vi "apply channel changes.vi"(8 "error in":errorcluster, 9 "TBM channel in":refnum<class "TBM channel.lvclass">, 10 "TBM channel in":refnum<class "TBM channel.lvclass">, 11 "Tag Bus Web Interface configuration in":refnum<class "Tag Bus Web Interface configuration.lvclass">) -> (0 "error out":errorcluster, 3 "Tag Bus Web Interface configuration out":refnum<class "Tag Bus Web Interface configuration.lvclass">)   [LabVIEW 2013, in "Tag Bus Web Interface configuration.lvclass"]
uses:
  Tag Bus Web Interface configuration.lvclass
  <vilib>/NI/Tag Bus Module Framework/channel/TBM channel.lvclass
  Tag Bus Web Interface configuration.lvclass/Tag Bus Web Interface configuration.ctl
  <vilib>/NI/Tag Bus/tag/tag descriptor.lvclass/tag descriptor.ctl
  <vilib>/NI/Tag Bus/tag/read tag name.vi
  <vilib>/NI/Tag Bus/tag/tag descriptor.lvclass
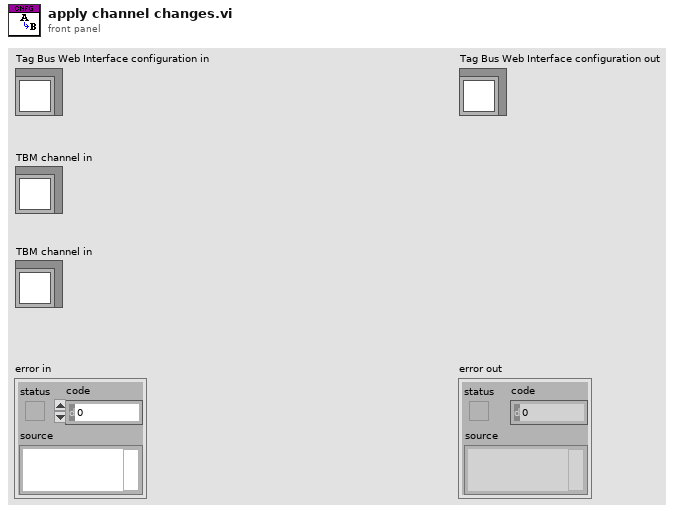
[diagram p1: front panel]
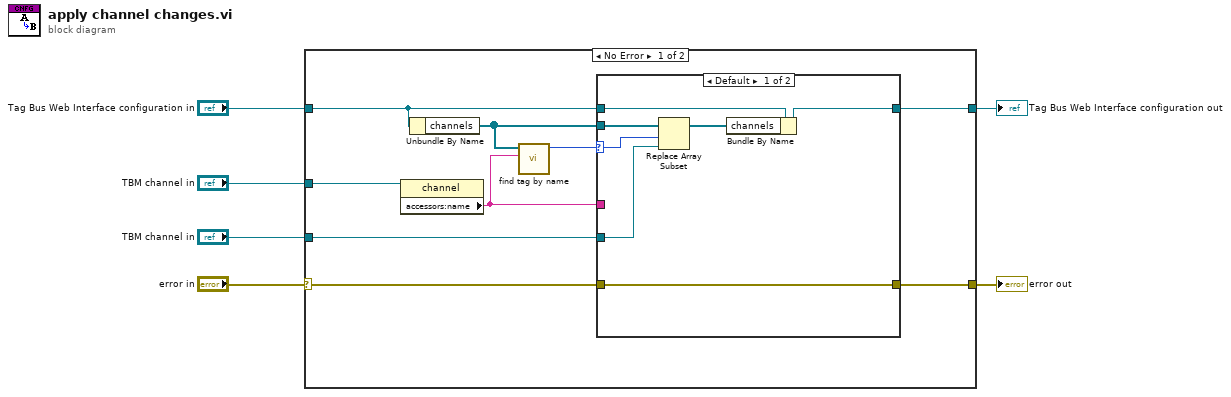
[diagram p0: block diagram]
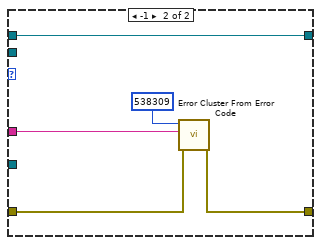
[diagram p2: hidden frame]
diagram:
  n1 = case shown="No Error" "error in" {
    selector: "error in" -> [w9 w29]
    tunnel: [w8 w29] -> w5
    tunnel: [w13 w28] -> w3
    tunnel: "Tag Bus Web Interface configuration in" -> [w14 w28]
    tunnel: "TBM channel in" -> [w15 _]
    tunnel: "TBM channel in" -> [w11 _]
    frame No Error {
      n2 = property class="channel"(reference=w15) -> ("accessors:name"=w10:string)  [unwired: 1 in, 2 out]
      n3 = Unbundle By Name(w14) -> ("channels"=w12:refnum<class "TBM channel.lvclass">[])
      n4 = call <vilib>:"find tag by name.vi"("name"=w10, "tags in"=w12) -> ("index"=w7:i32)  [unwired: 9 in]
      n5 = case shown="Default" w7 {
        selector: w7 -> [w20 _]
        tunnel: w14 -> [w22 w27]
        tunnel: [w19 w27] -> w13
        tunnel: w12 -> [w21 _]
        tunnel: w11 -> [w17 _]
        tunnel: w10 -> [_ w25]
        tunnel: w9 -> [w16 w24]
        tunnel: [w16 w23] -> w8
        frame Default {
          n6 = Replace Array Subset(array=w21, new element=w17, index=w20) -> (w18:refnum<class "TBM channel.lvclass">[])
          n7 = Bundle By Name(cluster=w22, "channels"=w18) -> (w19:refnum<class "Tag Bus Web Interface configuration.lvclass">)
        }
        frame -1 {
          n8 = call <vilib>:"Error Cluster From Error Code.vi"("error in (no error)"=w24, "error message (\"\")"=w25, "error code (0)"=538309) -> ("error out"=w23:errorcluster)  [unwired: 6 in]
        }
      }
    }
    frame Error {
    }
  }
  "error out" <- w5
  "Tag Bus Web Interface configuration out" <- w3
